vi "RSZVB Get Sweep Segment Spur Avoid.vi"(8 "error in (no error)":errorcluster {"code" format="%.0x"}, 9 "Segment (1)":i32=1, 10 "Channel (1)":i32=1, 11 "VISA session":refnum<visa-resource-name>) -> (0 "error out":errorcluster {"code" format="%.0x"}, 2 "Spur Avoid":i32, 3 "dup VISA session":refnum<visa-resource-name>)   [LabVIEW 2011]
doc: "This VI returns the position of the local oscillator frequency LO relative to the RF frequency (sideband, Spur Avoid) in sweep segment no. <Seg>. \n\nRemote-control command(s):\n[SENSe<Ch>:]SEGMent<Seg>:SBANd"
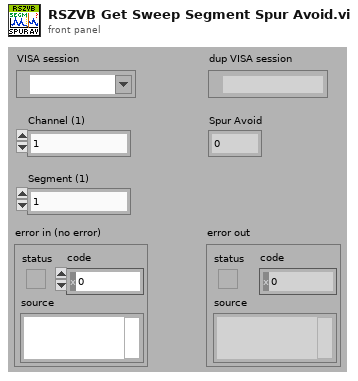
[diagram p1: front panel]
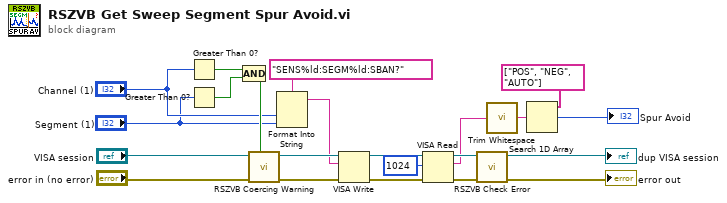
[diagram p0: block diagram]
diagram:
  n1 = Greater Than 0?(x="Channel (1)") -> (x > 0?=w17:bool)
  n2 = Greater Than 0?(x="Segment (1)") -> (x > 0?=w16:bool)
  n3 = Compound Arithmetic op=AND(w17, w16) -> (w19:bool)
  n4 = call "RSZVB Coercing Warning.vi"("In Range?"=w19, "error in (no error)"="error in (no error)", "VISA session"="VISA session") -> ("error out"=w20:errorcluster, "dup VISA session"=w21:refnum<visa-resource-name>)  [unwired: 7 in]
  n5 = Format Into String(format string="SENS%ld:SEGM%ld:SBAN?", "Channel (1)", "Segment (1)") -> (resulting string=w18:string)  [unwired: 2 in, 1 out]
  n6 = VISA Write(VISA resource name=w21, write buffer=w18, error in (no error)=w20) -> (VISA resource name out=w9:refnum<visa-resource-name>, error out=w8:errorcluster)  [unwired: 1 out]
  n7 = VISA Read(VISA resource name=w9, byte count=u32 1024 ("byte count (0)"), error in (no error)=w8) -> (VISA resource name out=w15:refnum<visa-resource-name>, read buffer=w11:string, error out=w14:errorcluster)  [unwired: 1 out]
  n8 = call "RSZVB Check Error.vi"("error in (no error)"=w14, "VISA session"=w15) -> ("error out"=→"error out":errorcluster, "dup VISA session"=→"dup VISA session":refnum<visa-resource-name>)  [unwired: 8 in]
  n9 = call <vilib>:"Trim Whitespace.vi"("string"=w11) -> ("trimmed string"=w13:string)  [unwired: 1 in]
  n10 = Search 1D Array(1D array=string[] ["POS", "NEG", "AUTO"] ("array 2"), element=w13) -> (index of element=→"Spur Avoid":i32)  [unwired: 1 in]
